vi "Check Log Status.vi"(8 "error in":errorcluster, 11 "Logger Interface in":refnum<class "Logger Interface.lvclass">) -> (0 "error out":errorcluster, 2 "Log file Size MB":dbl, 3 "Logger Interface out":refnum<class "Logger Interface.lvclass">, 4 "Hard Drive Space Used (%)":dbl, 5 "current filename":path)   [LabVIEW 2020, in "Frame Logging.lvlib" / "Logger Interface.lvclass"]
uses:
  Logger Interface.lvclass
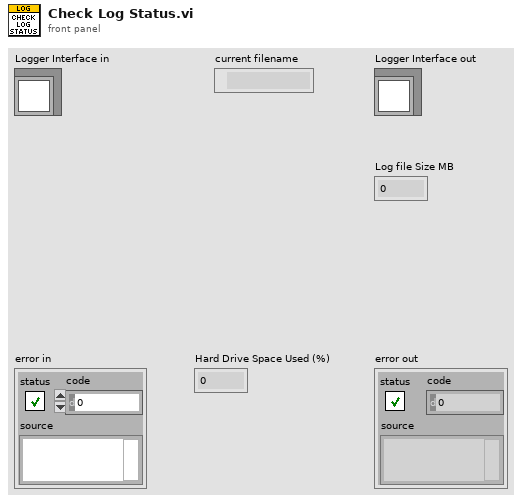
[diagram p1: front panel]
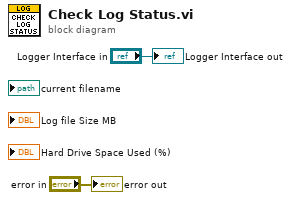
[diagram p0: block diagram]
diagram:
  "error out" <- "error in"
  "Logger Interface out" <- "Logger Interface in"
